vi "Stream Four Probe - Debug.vi"   [LabVIEW 2019]
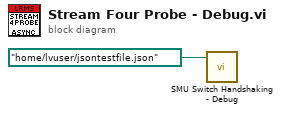
[diagram p0: block diagram]
diagram:
  n1 = call "SMU Switch Handshaking - Debug.vi"("file path (use dialog)"=path "/home/lvuser/jsontestfile.json") -> ()  [unwired: 10 in, 1 out]
